vi "ILC Tracking.vi"(6 "PID Cluster":T4={"L1 to L4 PID Cluster"={"L1 PID Gains"={"Kp"=0.005, "Kd"=0.5, "Ki"=0.0005}, "L2 PID Gains"={"Kp"=0.01, "Kd"=1.0, "Ki"=0.005}, "L3 PID Gains"={"Kp"=0.05, "Kd"=1.0, "Ki"=0.0005}, "L4 PID Gains"={"Kp"=0.1, "Kd"=0.1, "Ki"=0.0005}}, "Stage PID Cluster"={"Stage Z PID"={"Kp"=0.0005, "Kd"=0.001, "Ki"=0.0}, "Stage Y PID"={"Kp"=0.0003, "Kd"=0.01, "Ki"=0.0}, "Stage X PID"={"Kp"=0.0003, "Kd"=0.01, "Ki"=0.0}}, "OCT Z PID Gains"={"Kp"=0.0003, "Kd"=0.0001, "Ki"=0.01}}, 7 "Input RUY Signals":T1, 8 "error in":errorcluster, 9 "Offset Home 2 RCM":dbl[](array[numeric])=[0.0, 0.0, 0.0, 0.0], 10 "Prev Posit Cmd":T3={"Prev L1 to L4 Posit"=[-0.5319, -0.035669172703475985, -2.0566170657346783, 0.9099264705882353], "Prev Stage Posit"=[6.002553885707208, 5.996566124542428, 5.995469940427586], "Prev OCT Z Posit"=-0.0}, 11 "FPGA VI Reference In":refnum<k20>) -> (0 "error out":errorcluster, 2 "Last Posit Cmd":T2={"Last L1 to L4 Posit"=[0.0, 0.0, 0.0, 0.0], "Last Stage Posit"=[6.0, 6.0, 6.0], "Last OCT Z Posit"=0.0}, 3 "FPGA VI Reference Out":refnum<k20>, 5 "Output RUY Signals":T1)   [LabVIEW 2016]
uses:
  <vilib>/Platform/TimedLoop/XDataNode/timing_clust.ctl
  <vilib>/Platform/TimedLoop/XDataNode/nitl_modes.ctl
  <vilib>/Platform/TimedLoop/XDataNode/wakeup.ctl
  Global Variables.vi
  <vilib>/platform/TimedLoop/XDataNode/XDataNode.xnode
  <vilib>/Platform/TimedLoop/XDataNode/XDNodeRunTimeDep.lvlib
  Library/KevinLibraryAll/labview/KevLib01.lvlib
panel:
  out "In Servo Loop":bool
  out "Loading Finished":bool
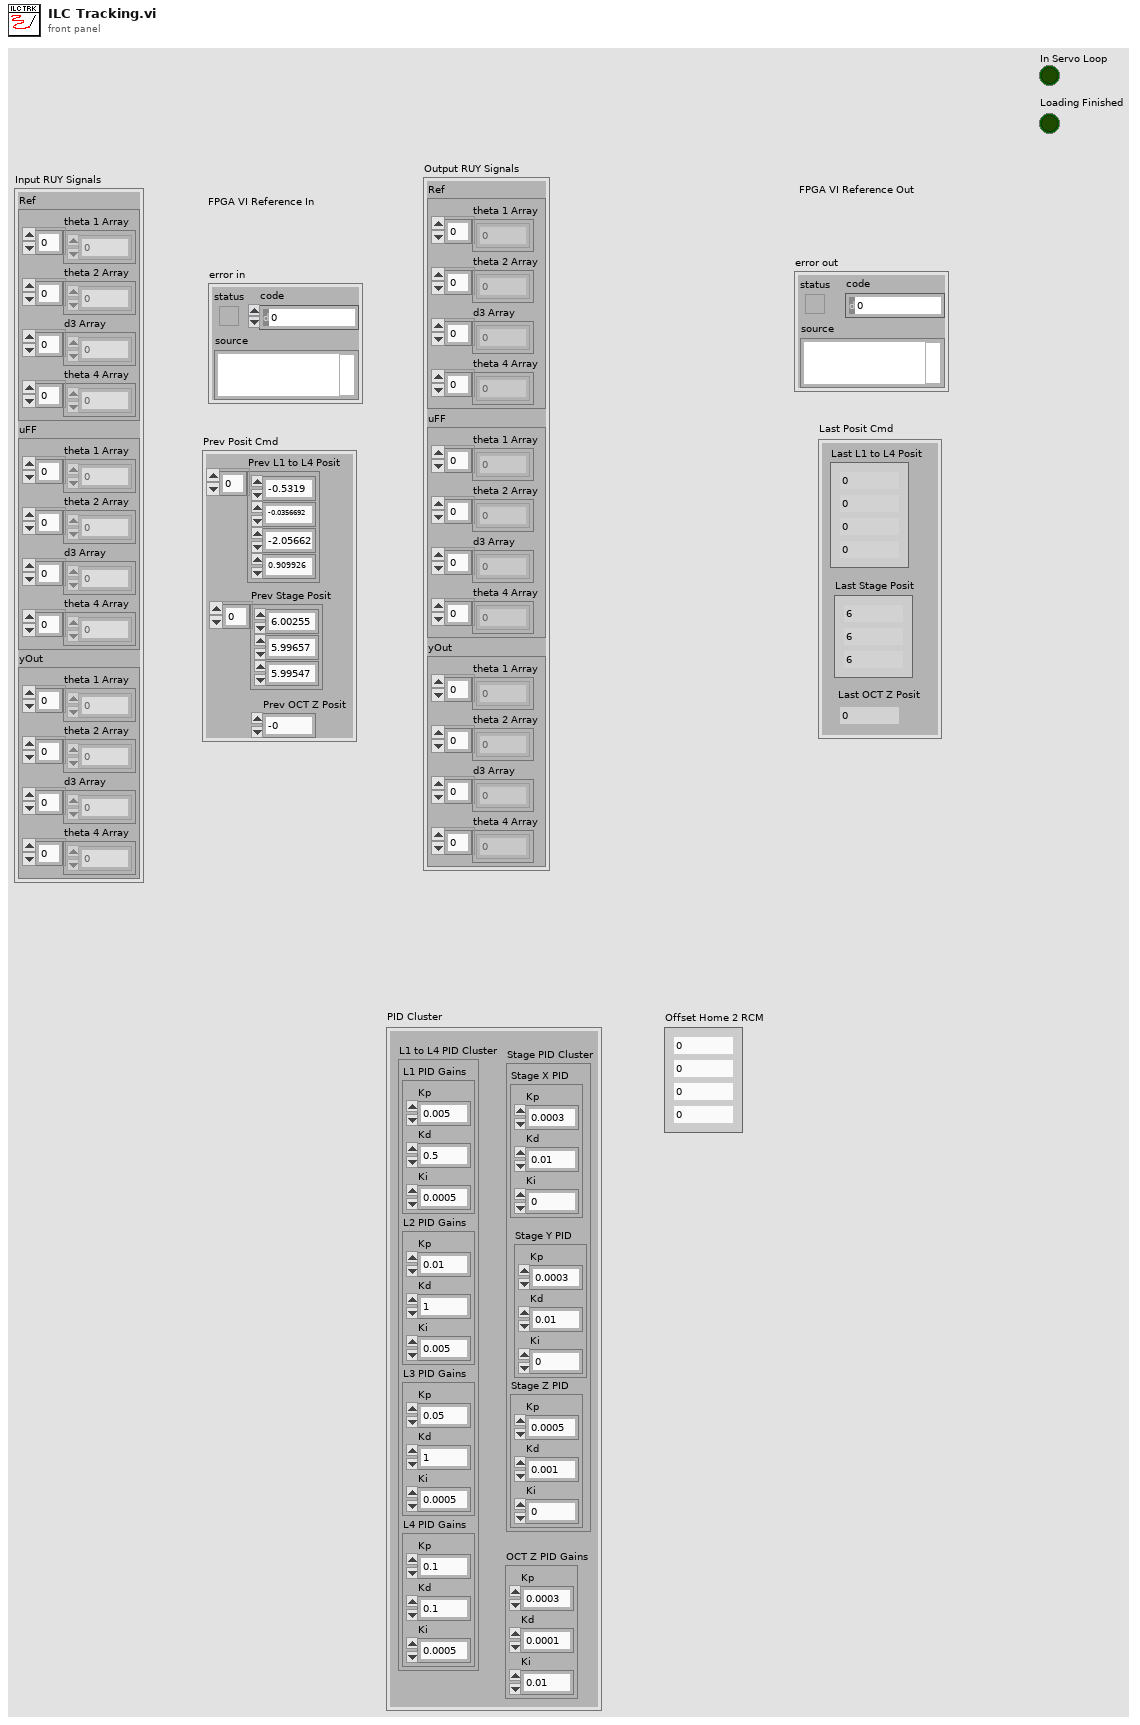
[diagram p1: front panel]
types:
  T1 = cluster{"Ref":cluster{"theta 1 Array":dbl[], "theta 2 Array":dbl[], "d3 Array":dbl[], "theta 4 Array":dbl[]}, "uFF":cluster{"theta 1 Array":dbl[], "theta 2 Array":dbl[], "d3 Array":dbl[], "theta 4 Array":dbl[]}, "yOut":cluster{"theta 1 Array":dbl[], "theta 2 Array":dbl[], "d3 Array":dbl[], "theta 4 Array":dbl[]}}
  T2 = cluster{"Last L1 to L4 Posit":dbl[], "Last Stage Posit":dbl[], "Last OCT Z Posit":dbl}
  T3 = cluster{"Prev L1 to L4 Posit":dbl[], "Prev Stage Posit":dbl[], "Prev OCT Z Posit":dbl}
  T4 = cluster{"L1 to L4 PID Cluster":cluster{"L1 PID Gains":cluster{"Kp":dbl, "Kd":dbl, "Ki":dbl}, "L2 PID Gains":cluster{"Kp":dbl, "Kd":dbl, "Ki":dbl}, "L3 PID Gains":cluster{"Kp":dbl, "Kd":dbl, "Ki":dbl}, "L4 PID Gains":cluster{"Kp":dbl, "Kd":dbl, "Ki":dbl}}, "Stage PID Cluster":cluster{"Stage Z PID":cluster{"Kp":dbl, "Kd":dbl, "Ki":dbl}, "Stage Y PID":cluster{"Kp":dbl, "Kd":dbl, "Ki":dbl}, "Stage X PID":cluster{"Kp":dbl, "Kd":dbl, "Ki":dbl}}, "OCT Z PID Gains":cluster{"Kp":dbl, "Kd":dbl, "Ki":dbl}}
  T5 = cluster{"Stop Vacuum":bool, "Vacuum Force":i8, "Max Limit [mmHg]":dbl, "Slide in":i8, "Irrigation?":bool}
  T6 = typedef "XDNodeRunTimeDep.lvlib/timing_clust.ctl" = cluster{"Expected End [f-1]":u64, "Actual End [f-1]":u64, "Finished Late? [f-1]":bool, "Expected End [i-1]":u64, "Actual End [i-1]":u64, "Finished Late? [i-1]":bool, "Expected Start [i]":u64, "Actual Start [i]":u64, "Expected Start [f]":u64, "Actual Start [f]":u64, "Source Name":string, "Structure Name":string, "Period":i64, "Deadline":i64, "Offset":i64, "Start":i64, "Priority":i32, "Timeout":i32, "Mode":T7, "Wakeup Reason":T8, "Error":errorcluster, "Source Type":string, "Secondary Source Type":string, "Global End Time":u64, "Global Start Time":u64, "Frame Duration":u64, "Iteration Duration":u64, "Assigned CPU":i32, "I/O Scan Engine Mode":u32}
  T7 = typedef "XDNodeRunTimeDep.lvlib/nitl_modes.ctl" = enum32{"No Change", "Process missed periods, maintain original phase", "Discard missed periods, maintain original phase", "Process missed periods, ignore original phase", "Discard missed periods, ignore original phase"}
  T8 = typedef "XDNodeRunTimeDep.lvlib/wakeup.ctl" = enum32{"Normal", "Aborted", "Asynchronous wakeup", "Timing source error", "Timed loop error", "Timeout"}
  T9 = cluster{"L1 PID Gains":cluster{"Kp":dbl, "Kd":dbl, "Ki":dbl}, "L2 PID Gains":cluster{"Kp":dbl, "Kd":dbl, "Ki":dbl}, "L3 PID Gains":cluster{"Kp":dbl, "Kd":dbl, "Ki":dbl}, "L4 PID Gains":cluster{"Kp":dbl, "Kd":dbl, "Ki":dbl}}
  T10 = cluster{"Stage Z PID":cluster{"Kp":dbl, "Kd":dbl, "Ki":dbl}, "Stage Y PID":cluster{"Kp":dbl, "Kd":dbl, "Ki":dbl}, "Stage X PID":cluster{"Kp":dbl, "Kd":dbl, "Ki":dbl}}
  T11 = cluster{"Accurus button":bool[], "Accurus engaged?":bool, "Vacuum Force":i32, "Accurus Ch. A Vout":dbl, "Accurus Ch. B Vout":dbl, "Irrigation engaged?":bool}
  T12 = cluster{"theta 1 Array":dbl[], "theta 2 Array":dbl[], "d3 Array":dbl[], "theta 4 Array":dbl[]}
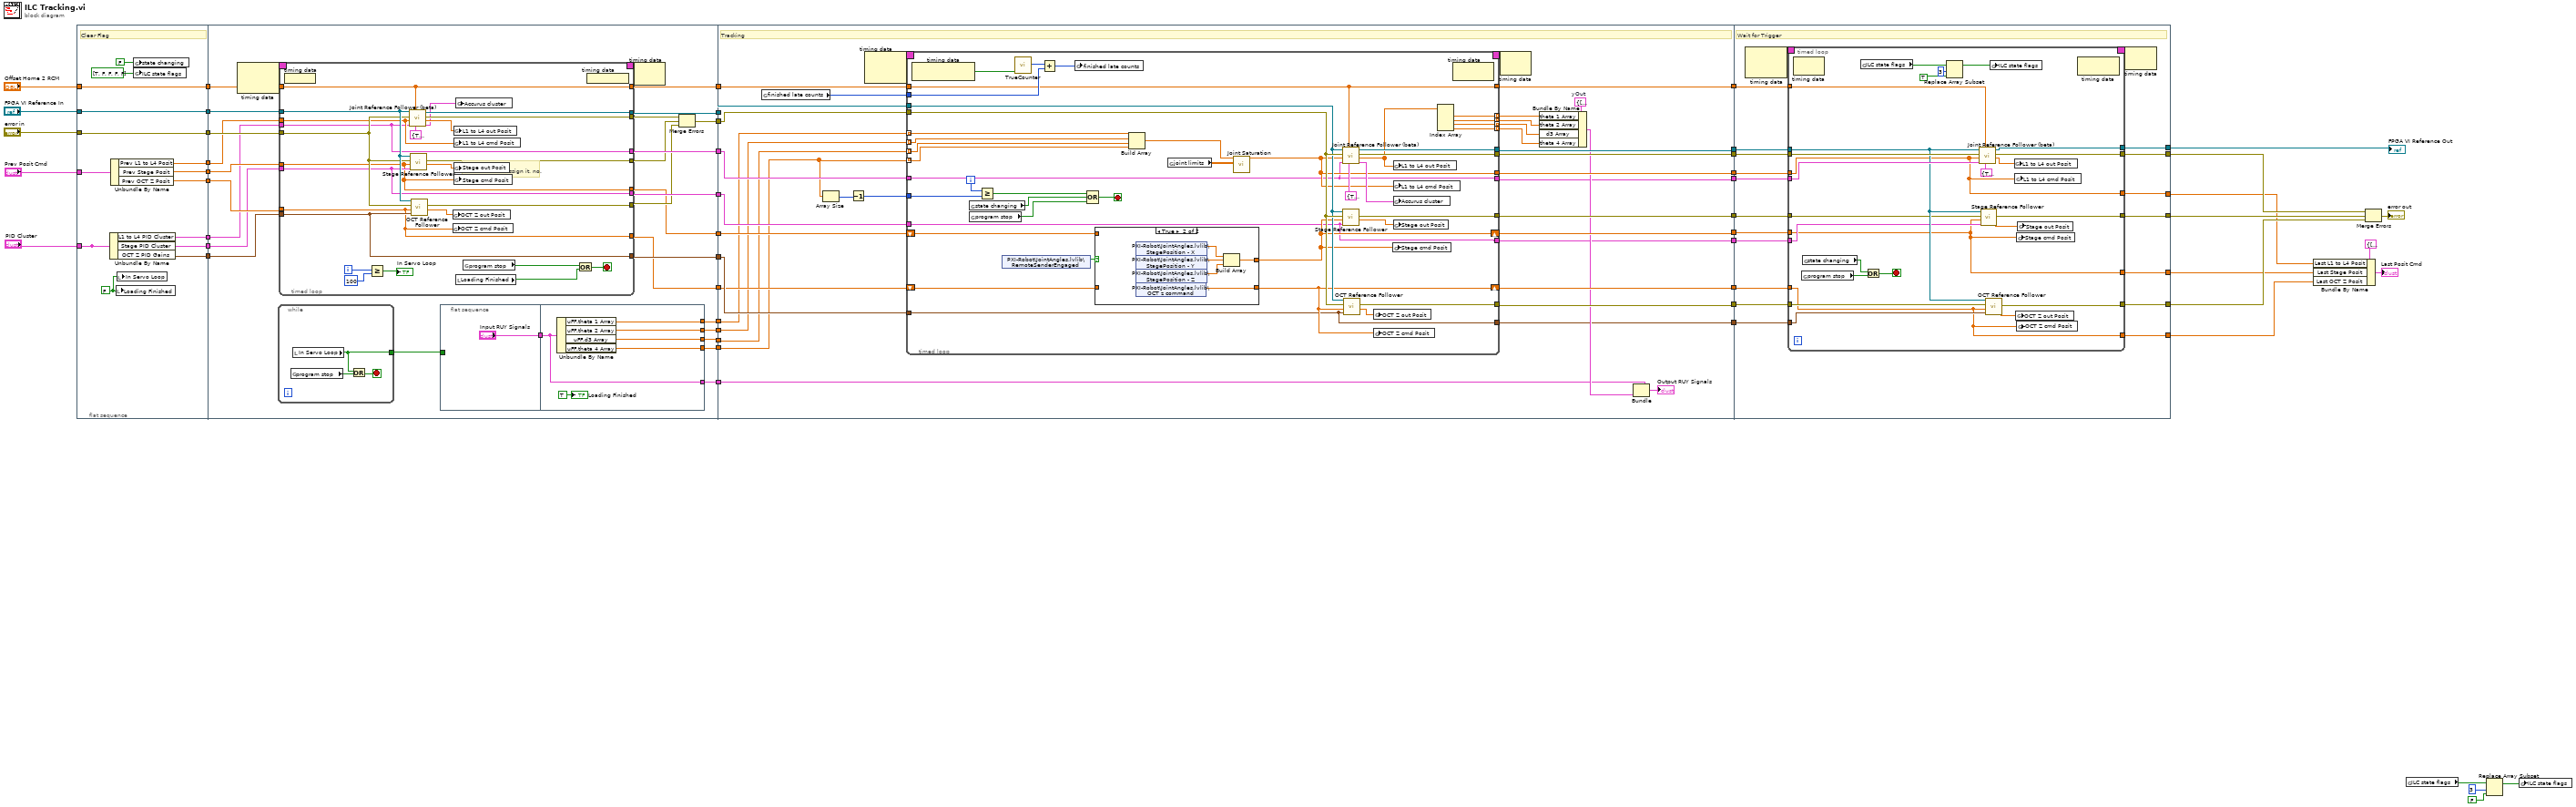
[diagram p0: block diagram]
diagram:
  n1 = flat-sequence {
    tunnel: [w66] -> w52
    tunnel: "FPGA VI Reference In" -> [w66]
    tunnel: "error in" -> [w65]
    tunnel: [w65] -> w49
    tunnel: "Prev Posit Cmd" -> [w64]
    tunnel: [w63] -> _
    tunnel: "PID Cluster" -> [w63]
    tunnel: [w62] -> w46
    tunnel: [w61] -> w45
    tunnel: [w60] -> w44
    tunnel: [w59] -> w43
    tunnel: [w58] -> w42
    tunnel: "Offset Home 2 RCM" -> [w58]
    tunnel: [w57] -> w37
    tunnel: [w55] -> w30
    tunnel: w52 -> [w95]
    tunnel: w49 -> [w94]
    tunnel: w46 -> [w93]
    tunnel: w45 -> [w92]
    tunnel: w44 -> [w91]
    tunnel: w43 -> [w90]
    tunnel: w42 -> [w89]
    tunnel: [w88] -> w40
    tunnel: [w87] -> w39
    tunnel: [w86] -> w38
    tunnel: w37 -> [w85]
    tunnel: [w84] -> w36
    tunnel: [w83] -> w35
    tunnel: [w82] -> w34
    tunnel: w30 -> [w81]
    tunnel: [w75] -> w29
    tunnel: [w74] -> w28
    tunnel: [w71] -> w23
    tunnel: [w70] -> w22
    tunnel: [w69] -> w21
    tunnel: [w68] -> w20
    tunnel: [w67] -> w19
    tunnel: w40 -> [w167]
    tunnel: w39 -> [w153]
    tunnel: w38 -> [w166]
    tunnel: w36 -> [w164]
    tunnel: w35 -> [w163]
    tunnel: w34 -> [w162]
    tunnel: w29 -> [w155]
    tunnel: w28 -> [w154]
    tunnel: w23 -> [w137]
    tunnel: w22 -> [w149]
    tunnel: w21 -> [w148]
    tunnel: w20 -> [w147]
    tunnel: w19 -> [w146]
    tunnel: [w161] -> w11
    tunnel: [w160] -> w10
    tunnel: [w159] -> w9
    tunnel: [w158] -> w8
    tunnel: [w150] -> w7
    tunnel: [w157] -> w6
    tunnel: [w156] -> w5
    tunnel: [w139] -> w4
    tunnel: [w138] -> w3
    tunnel: [w136] -> w2
    tunnel: [w135] -> w1
    tunnel: w11 -> [w239]
    tunnel: w10 -> [w238]
    tunnel: w9 -> [w232]
    tunnel: w8 -> [w233]
    tunnel: w6 -> [w235]
    tunnel: w5 -> [w234]
    tunnel: w4 -> [w240]
    tunnel: w3 -> [w236]
    tunnel: w1 -> [w231]
    tunnel: w2 -> [w230]
    tunnel: [w229] -> w16
    tunnel: [w228] -> w17
    tunnel: [w227] -> w18
    tunnel: [w226] -> w15
    tunnel: [w225] -> w14
    tunnel: [w224] -> w13
    tunnel: [w223] -> w12
    tunnel: w7 -> [w237]
    frame #0 {
      w56 = FALSE ("Loading Finished")
      # "Clear Flag"
      n2 = Unbundle By Name(w63) -> ("L1 to L4 PID Cluster"=w59:T9, "Stage PID Cluster"=w57:T10, "OCT Z PID Gains"=w62:cluster{"Kp":dbl, "Kd":dbl, "Ki":dbl})
      n3 = Unbundle By Name(w64) -> ("Prev L1 to L4 Posit"=w55:dbl[], "Prev Stage Posit"=w61:dbl[], "Prev OCT Z Posit"=w60:dbl)
      n4 = local write "Loading Finished"(w56) -> ()
      n5 = local write "In Servo Loop"(w56) -> ()
      n6 = global write "Global Variables.vi" "state changing"(FALSE ("state changing")) -> ()
      n7 = global write "Global Variables.vi" "ILC state flags"(bool[] [TRUE, FALSE, FALSE, FALSE, FALSE]) -> ()
    }
    frame #1 {
      # "terminate loop\nwhen it. no. > assign it. no."
      n8 = node-c288() -> (w80:T6)  [unwired: 2 in]
      n9 = while {
        tunnel: [w96] -> w73
        stop <- w98 stop-if-true
        n10 = global read "Global Variables.vi" "program stop"() -> (w97:bool)
        n11 = local read "In Servo Loop"() -> (w96:bool)
        n12 = Or(x=w96, y=w97) -> (x .or. y?=w98:bool)
      }
      n13 = timed-loop {
        timing: w80 -> [_]
        timing-out: [_] -> w79
        tunnel: [w107] -> w75
        tunnel: [w106] -> w74
        tunnel: [w123] -> w88
        tunnel: [w122] -> w78
        tunnel: [w121] -> w77
        tunnel: [w120] -> w76
        tunnel: w95 -> [w119]
        tunnel: w94 -> [w118]
        tunnel: w93 -> [w115]
        tunnel: w81 -> [w117]
        tunnel: w92 -> [w107]
        tunnel: w91 -> [w106]
        tunnel: w90 -> [w113]
        tunnel: w89 -> [w116]
        tunnel: [w116] -> w87
        tunnel: w85 -> [w114]
        tunnel: [w115] -> w82
        tunnel: [w114] -> w83
        tunnel: [w113] -> w84
        i -> [w112]
        stop <- w129 stop-if-true
        n14 = node-c288 ("Output Node")() -> ()  [unwired: 1 in]
        n15 = Greater Or Equal?(x=w112, y=100) -> (x >= y?=→"In Servo Loop":bool)
        n16 = call "Joint Reference Follower (beta).vi"("Accurus Ctrl Cluster"=T5 {"Stop Vacuum"=TRUE, "Vacuum Force"=0, "Max Limit [mmHg]"=600.0, "Slide in"=0, "Irrigation?"=TRUE}, "Offset Home2RCM [deg/mm]"=w116, "PID Ctrl Cluster"=w113, "Ref Array [deg/mm]"=w117, "error in"=w118, "FPGA VI Reference In"=w119) -> ("Accurus Output Cluster"=w108:T11, "Output Posit Array [deg/mm]"=w126:dbl[], "error out"=w122:errorcluster, "FPGA VI Reference Out"=w123:refnum<k20>)  [unwired: 2 in]
        n17 = call "Stage Reference Follower.vi"("Stage PID Cluster"=w114, "Stage cmd Posit [mm]"=w107, "error in"=w118, "FPGA VI Reference In"=w119) -> ("Stage out Posit [mm]"=w125:dbl[], "error out"=w121:errorcluster)  [unwired: 5 in, 1 out]
        n18 = call "OCT Reference Follower.vi"("OCT Z PID Gains"=w115, "OCT  Z cmd Posit [mm]"=w106, "error in"=w118, "FPGA VI Reference In"=w119) -> ("OCT  Z out Posit [mm]"=w124:dbl, "error out"=w120:errorcluster)  [unwired: 5 in, 1 out]
        n19 = global write "Global Variables.vi" "OCT Z out Posit"(w124) -> ()
        n20 = global write "Global Variables.vi" "OCT Z cmd Posit"(w106) -> ()
        n21 = global write "Global Variables.vi" "L1 to L4 out Posit"(w126) -> ()
        n22 = global write "Global Variables.vi" "L1 to L4 cmd Posit"(w117) -> ()
        n23 = global write "Global Variables.vi" "Stage out Posit"(w125) -> ()
        n24 = global write "Global Variables.vi" "Stage cmd Posit"(w107) -> ()
        n25 = global write "Global Variables.vi" "Accurus cluster"(w108) -> ()
        n26 = local read "Loading Finished"() -> (w128:bool)
        n27 = global read "Global Variables.vi" "program stop"() -> (w127:bool)
        n28 = Or(x=w127, y=w128) -> (x .or. y?=w129:bool)
        n29 = node-c288() -> ()  [unwired: 1 out]
      }
      n30 = flat-sequence {
        tunnel: w73 -> [_]
        tunnel: ["Input RUY Signals"] -> w72
        tunnel: w72 -> [w100]
        tunnel: [w104] -> w70
        tunnel: [w103] -> w69
        tunnel: [w102] -> w68
        tunnel: [w101] -> w67
        tunnel: [w100] -> w71
        frame #0 {
        }
        frame #1 {
          n31 = Unbundle By Name(w100) -> ("uFF.theta 1 Array"=w104:dbl[], "uFF.theta 2 Array"=w103:dbl[], "uFF.d3 Array"=w102:dbl[], "uFF.theta 4 Array"=w101:dbl[])
          "Loading Finished" <- TRUE ("Loading Finished")
        }
      }
      n32 = node-c288(w79) -> ()  [unwired: 1 out]
      n33 = Merge Errors(w78, w77, w76) -> (w86:errorcluster)
    }
    frame #2 {
      w144 = T12 {"theta 1 Array"=[], "theta 2 Array"=[], "d3 Array"=[], "theta 4 Array"=[]}  # yOut
      # "Tracking"
      n34 = global read "Global Variables.vi" "finished late counts"() -> (w165:u16)
      n35 = Array Size(array=w146) -> (size(s)=w152:i32)
      n36 = Decrement(x=w152) -> (x-1=w151:i32)
      n37 = node-c288() -> (w169:T6)  [unwired: 2 in]
      n38 = timed-loop {
        timing: w169 -> [_]
        timing-out: [_] -> w168
        tunnel: w149 -> [w187] mode=indexing
        tunnel: w148 -> [w186] mode=indexing
        tunnel: w147 -> [w185] mode=indexing
        tunnel: w167 -> [w208]
        tunnel: w153 -> [w173]
        tunnel: w166 -> [w209]
        tunnel: [w210] -> w161
        tunnel: w164 -> [w172]
        tunnel: w165 -> [w204]
        tunnel: w163 -> [w171]
        tunnel: w162 -> [w170]
        shift-right: [w181] -> w157
        shift-left: w155 -> [w200]
        shift-right: [w180] -> w156
        shift-left: w154 -> [w199]
        tunnel: [w198] -> w159
        tunnel: [w197] -> w158
        tunnel: [w196] -> w160
        tunnel: w151 -> [w193]
        tunnel: w146 -> [w184] mode=indexing
        tunnel: [w182] -> w150
        tunnel: [w177] -> w143 mode=indexing
        tunnel: [w176] -> w142 mode=indexing
        tunnel: [w175] -> w141 mode=indexing
        tunnel: [w174] -> w140 mode=indexing
        tunnel: [w173] -> w139
        tunnel: [w172] -> w138
        tunnel: [w171] -> w135
        tunnel: [w170] -> w136
        i -> [w188]
        stop <- w189 stop-if-true
        n39 = node-c288() -> (w207:bool)  [unwired: 1 in]
        n40 = global read "Global Variables.vi" "state changing"() -> (w191:bool)
        n41 = global read "Global Variables.vi" "program stop"() -> (w190:bool)
        n42 = Greater Or Equal?(x=w188, y=w193) -> (x >= y?=w192:bool)
        n43 = shared-variable "PXI-Robot\\JointAngles.lvlib\\RemoteSenderEngaged"() -> (w203:bool)  [unwired: 1 in, 1 out]
        n44 = call "TrueCounter.vi"("True?"=w207) -> ("True Count"=w205:u16)  [unwired: 10 in]
        n45 = Add(x=w205, y=w204) -> (x+y=w206:u16)
        n46 = global write "Global Variables.vi" "finished late counts"(w206) -> ()
        n47 = Compound Arithmetic op=OR(w192, w191, w190) -> (w189:bool)
        n48 = case shown="True" w203 {
          tunnel: [w212 w214] -> w181
          tunnel: [w211 w213] -> w180
          tunnel: w200 -> [w212 _]
          tunnel: w199 -> [w211 _]
          frame False {
            # "Hold Position if not Engaged"
          }
          frame True {
            n49 = shared-variable "PXI-Robot\\JointAngles.lvlib\\StagePosition - X"() -> (w217:dbl)  [unwired: 1 in, 1 out]
            n50 = shared-variable "PXI-Robot\\JointAngles.lvlib\\StagePosition - Y"() -> (w216:dbl)  [unwired: 1 in, 1 out]
            n51 = shared-variable "PXI-Robot\\JointAngles.lvlib\\StagePosition - Z"() -> (w215:dbl)  [unwired: 1 in, 1 out]
            n52 = shared-variable "PXI-Robot\\JointAngles.lvlib\\OCT z command"() -> (w213:dbl)  [unwired: 1 in, 1 out]
            n53 = Build Array(w217, w216, w215) -> (w214:dbl[])
          }
        }
        n54 = Build Array(w187, w186, w185, w184) -> (w183:dbl[])
        n55 = global read "Global Variables.vi" "joint limits"() -> (w179:dbl[][])
        n56 = call "Joint Saturation.vi"("Joint Bounds [Deg/mm]"=w179, "Ref Array [Deg/mm]"=w183) -> ("Sat Ref Array [Deg/mm]"=w182:dbl[])  [unwired: 9 in]
        n57 = call "Joint Reference Follower (beta).vi"("Accurus Ctrl Cluster"=T5 {"Stop Vacuum"=TRUE, "Vacuum Force"=0, "Max Limit [mmHg]"=600.0, "Slide in"=0, "Irrigation?"=FALSE}, "Offset Home2RCM [deg/mm]"=w173, "PID Ctrl Cluster"=w172, "Ref Array [deg/mm]"=w182, "error in"=w209, "FPGA VI Reference In"=w208) -> ("Accurus Output Cluster"=w195:T11, "Output Posit Array [deg/mm]"=w178:dbl[], "error out"=w196:errorcluster, "FPGA VI Reference Out"=w210:refnum<k20>)  [unwired: 2 in]
        n58 = call "Stage Reference Follower.vi"("Stage PID Cluster"=w171, "Stage cmd Posit [mm]"=w181, "error in"=w209, "FPGA VI Reference In"=w208) -> ("Stage out Posit [mm]"=w202:dbl[], "error out"=w198:errorcluster)  [unwired: 5 in, 1 out]
        n59 = call "OCT Reference Follower.vi"("OCT Z PID Gains"=w170, "OCT  Z cmd Posit [mm]"=w180, "error in"=w209, "FPGA VI Reference In"=w208) -> ("OCT  Z out Posit [mm]"=w201:dbl, "error out"=w197:errorcluster)  [unwired: 5 in, 1 out]
        n60 = global write "Global Variables.vi" "OCT Z out Posit"(w201) -> ()
        n61 = global write "Global Variables.vi" "OCT Z cmd Posit"(w180) -> ()
        n62 = global write "Global Variables.vi" "Stage cmd Posit"(w181) -> ()
        n63 = global write "Global Variables.vi" "L1 to L4 out Posit"(w178) -> ()
        n64 = global write "Global Variables.vi" "L1 to L4 cmd Posit"(w182) -> ()
        n65 = global write "Global Variables.vi" "Accurus cluster"(w195) -> ()
        n66 = global write "Global Variables.vi" "Stage out Posit"(w202) -> ()
        n67 = Index Array(array=w178) -> (element #1=w177:dbl, element #2=w176:dbl, element #3=w175:dbl, element #4=w174:dbl)  [unwired: 4 in]
        n68 = node-c288() -> ()  [unwired: 1 in, 1 out]
      }
      n69 = node-c288(w168) -> ()  [unwired: 1 out]
      n70 = Bundle By Name(cluster=w144, "theta 1 Array"=w143, "theta 2 Array"=w142, "d3 Array"=w141, "theta 4 Array"=w140) -> (w145:T12)
      n71 = Bundle(cluster=w137, "yOut"=w145) -> (→"Output RUY Signals":T1)  [unwired: 2 in]
    }
    frame #3 {
      # "Wait for Trigger"
      n72 = node-c288() -> (w242:T6)  [unwired: 2 in]
      n73 = timed-loop {
        timing: w242 -> [_]
        timing-out: [_] -> w241
        tunnel: w240 -> [w258]
        tunnel: w239 -> [w254]
        tunnel: w238 -> [w257]
        tunnel: w237 -> [w245]
        tunnel: w236 -> [w256]
        tunnel: w235 -> [w244]
        tunnel: w234 -> [w243]
        tunnel: w233 -> [w255]
        tunnel: w232 -> [w253]
        tunnel: w231 -> [w252]
        tunnel: w230 -> [w251]
        tunnel: [w249] -> w229
        tunnel: [w248] -> w228
        tunnel: [w247] -> w227
        tunnel: [w246] -> w226
        tunnel: [w245] -> w225
        tunnel: [w244] -> w224
        tunnel: [w243] -> w223
        stop <- w250 stop-if-true
        n74 = node-c288() -> ()  [unwired: 1 in, 1 out]
        n75 = global read "Global Variables.vi" "program stop"() -> (w264:bool)
        n76 = global read "Global Variables.vi" "state changing"() -> (w260:bool)
        n77 = global read "Global Variables.vi" "ILC state flags"() -> (w263:bool[])
        n78 = Or(x=w260, y=w264) -> (x .or. y?=w250:bool)
        n79 = Replace Array Subset(array=w263, new element=TRUE ("new element/subarray"), index=3) -> (w261:bool[])
        n80 = call "Joint Reference Follower (beta).vi"("Accurus Ctrl Cluster"=T5 {"Stop Vacuum"=TRUE, "Vacuum Force"=0, "Max Limit [mmHg]"=600.0, "Slide in"=0, "Irrigation?"=FALSE}, "Offset Home2RCM [deg/mm]"=w258, "PID Ctrl Cluster"=w256, "Ref Array [deg/mm]"=w245, "error in"=w257, "FPGA VI Reference In"=w254) -> ("Output Posit Array [deg/mm]"=w268:dbl[], "error out"=w249:errorcluster, "FPGA VI Reference Out"=w246:refnum<k20>)  [unwired: 2 in, 1 out]
        n81 = call "Stage Reference Follower.vi"("Stage PID Cluster"=w252, "Stage cmd Posit [mm]"=w244, "error in"=w253, "FPGA VI Reference In"=w254) -> ("Stage out Posit [mm]"=w267:dbl[], "error out"=w248:errorcluster)  [unwired: 5 in, 1 out]
        n82 = call "OCT Reference Follower.vi"("OCT Z PID Gains"=w251, "OCT  Z cmd Posit [mm]"=w243, "error in"=w255, "FPGA VI Reference In"=w254) -> ("OCT  Z out Posit [mm]"=w266:dbl, "error out"=w247:errorcluster)  [unwired: 5 in, 1 out]
        n83 = global write "Global Variables.vi" "ILC state flags"(w261) -> ()
        n84 = global write "Global Variables.vi" "L1 to L4 out Posit"(w268) -> ()
        n85 = global write "Global Variables.vi" "L1 to L4 cmd Posit"(w245) -> ()
        n86 = global write "Global Variables.vi" "OCT Z out Posit"(w266) -> ()
        n87 = global write "Global Variables.vi" "Stage cmd Posit"(w244) -> ()
        n88 = global write "Global Variables.vi" "OCT Z cmd Posit"(w243) -> ()
        n89 = global write "Global Variables.vi" "Stage out Posit"(w267) -> ()
        n90 = node-c288() -> ()  [unwired: 1 in, 1 out]
      }
      n91 = node-c288(w241) -> ()  [unwired: 1 out]
    }
  }
  n92 = Bundle By Name(cluster=T2 {"Last L1 to L4 Posit"=[0.0, 0.0, 0.0, 0.0], "Last Stage Posit"=[6.0, 6.0, 6.0], "Last OCT Z Posit"=0.0} ("Last Posit Cluster 2"), "Last L1 to L4 Posit"=w14, "Last Stage Posit"=w13, "Last OCT Z Posit"=w12) -> (→"Last Posit Cmd":T2)
  n93 = Merge Errors(w16, w17, w18) -> (→"error out":errorcluster)
  n94 = global read "Global Variables.vi" "ILC state flags"() -> (w25:bool[])
  n95 = Replace Array Subset(array=w25, new element=FALSE ("new element/subarray"), index=3) -> (w24:bool[])
  n96 = global write "Global Variables.vi" "ILC state flags"(w24) -> ()
  "FPGA VI Reference Out" <- w15
